vi "VHM-connectionSettings.vi"(8 "error in (no error)":errorcluster, 10 "connection settings":T1={"Com"="", "baud rate (9600)"=38400} {"baud rate (9600)" items=["75"=75, "110"=110, "134"=134, "150"=150, "300"=300, "600"=600, "1200"=1200, "1800"=1800, "2400"=2400, "4800"=4800, "7200"=7200, "9600"=9600, "14400"=14400, "19200"=19200, "28800"=28800, "38400"=38400, "56000"=56000, "57600"=57600, "115200"=115200, "128000"=128000, "230400"=230400]}, 11 "VHM-VNA_Hardware_Manager in":refnum<class "VHM-VNA_Hardware_Manager.lvclass">) -> (0 "error out":errorcluster, 3 "VHM-VNA_Hardware_Manager out":refnum<class "VHM-VNA_Hardware_Manager.lvclass">)   [LabVIEW 2020, in "VHM-VNA_Hardware_Manager.lvlib" / "VHM-VNA_Hardware_Manager.lvclass"]
uses:
  VHM-VNA_Hardware_Manager.lvclass
  classes/vna-drivers/liteVNA/VD-connection_settings.ctl
  classes/hardware-protocol/serial/HP-S-baudrate.ctl
  VHM-VNA_Hardware_Manager.lvclass/VHM-VNA_Hardware_Manager.ctl
  classes/vna-drivers/liteVNA/VD-LV-LiteVNA.lvclass
  classes/hardware-protocol/serial/HP-S-Serial.lvclass
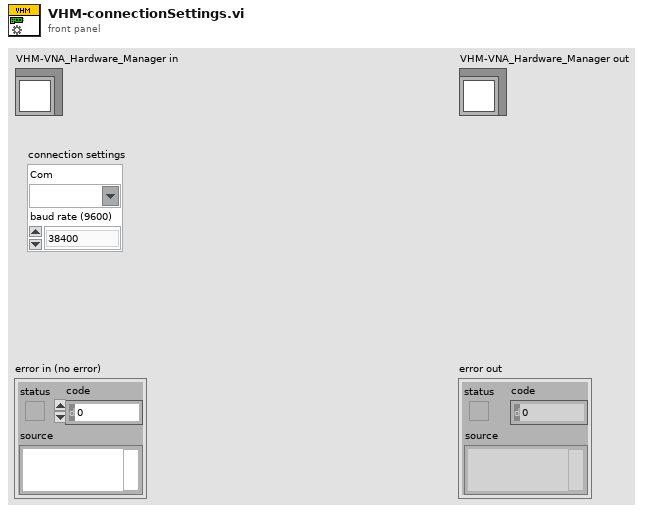
[diagram p1: front panel]
types:
  T1 = typedef "VD-LV-LiteVNA.lvclass/VD-connection_settings.ctl" = cluster{"Com":refnum<visa-resource-name>, "baud rate (9600)":T2}
  T2 = typedef "HP-S-Serial.lvclass/HP-S-baudrate.ctl" = u32
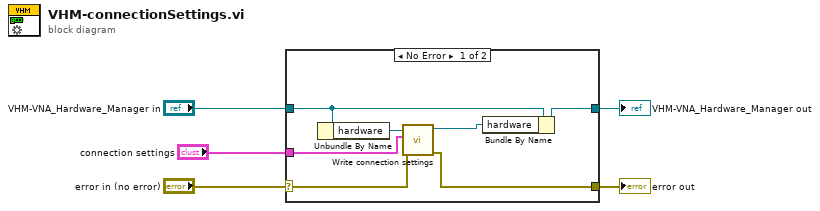
[diagram p0: block diagram]
diagram:
  n1 = case shown="No Error" "error in (no error)" {
    selector: "error in (no error)" -> [w7 w14]
    tunnel: [w6 w14] -> w4
    tunnel: [w11 w13] -> w2
    tunnel: "VHM-VNA_Hardware_Manager in" -> [w12 w13]
    tunnel: "connection settings" -> [w8 _]
    frame No Error {
      n2 = Unbundle By Name(w12) -> ("hardware"=w10:refnum<class "VD-LV-LiteVNA.lvclass">)
      n3 = call-dynamic "Write connection settings.vi"("error in (no error)"=w7, "connection settings"=w8, "VD-LV-LiteVNA in"=w10) -> ("error out"=w6:errorcluster, "VD-LV-LiteVNA out"=w9:refnum<class "VD-LV-LiteVNA.lvclass">)  [unwired: 7 in]
      n4 = Bundle By Name(cluster=w12, "hardware"=w9) -> (w11:refnum<class "VHM-VNA_Hardware_Manager.lvclass">)
    }
    frame Error {
    }
  }
  "error out" <- w4
  "VHM-VNA_Hardware_Manager out" <- w2
